vi "DIO Read Bank.vi"(6 "DI.DMA_ENA":T1, 8 "DI.DMA_CNTR":u16=5, 10 "DATA IN":fxp<+,20,20> format="%.0b", 11 "DMA FIFO IN":refnum<k21>="DI") -> (0 "DI.DMA_IDL":bool, 2 "DIO.A_0:15.IN":fxp<+,20,20> format="%.0b")   [LabVIEW 2019]
uses:
  Utilities/Start Boolean.ctl
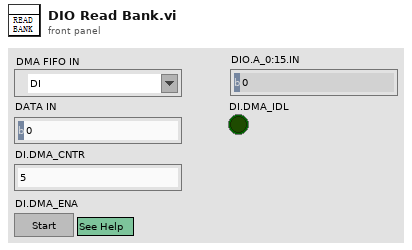
[diagram p1: front panel]
types:
  T1 = typedef "Start Boolean.ctl" = bool
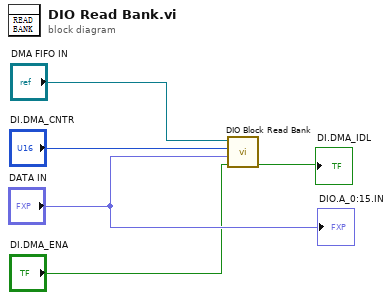
[diagram p0: block diagram]
diagram:
  n1 = call "DIO Block Read Bank.vi"("DI.DMA_ENA"="DI.DMA_ENA", "DATA IN"="DATA IN", "DI.DMA_CNTR"="DI.DMA_CNTR", "DMA FIFO In"="DMA FIFO IN") -> ("DI.DMA_IDL"=→"DI.DMA_IDL":bool)  [unwired: 7 in]
  "DIO.A_0:15.IN" <- "DATA IN"
